vi "Format Priority String.vi"(11 "Priority":T1(ring)) -> (3 "Priority String":string)   [LabVIEW 2020, in "VI Properties Editor.lvlib"]
doc: "Formats the reentrancy, priority, and preferred execution system properties into strings to be displayed."
uses:
  VI Properties Editor.lvlib
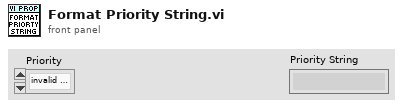
[diagram p1: front panel]
types:
  T1 = enum32{"invalid priority", "background priority", "normal priority", "above normal priority", "high priority", "time critical priority", "subroutine"}
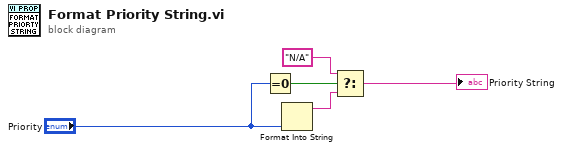
[diagram p0: block diagram]
diagram:
  n1 = Equal To 0?(x="Priority") -> (x = 0?=w4:bool)
  n2 = Format Into String("Priority") -> (resulting string=w2:string)  [unwired: 3 in, 1 out]
  n3 = Select(t="N/A", s=w4, f=w2) -> (s? t:f=→"Priority String":string)
